vi "dsbsc1.vi"() -> ()   [LabVIEW 2018]
uses:
  <vilib>/express/express analysis/Spectral/Block/exnSpectralBlock spectral measurements RMS poly.vi
  <vilib>/express/express analysis/Spectral/Block/exnSpectralBlock spectral measurements RMS DDT.vi
  <vilib>/express/express analysis/Spectral/XNode/ExpressSpectralMeasurementsBlockNode.xnode
panel:
  out "Waveform Graph 4":dynamicdata(graph)
  out "Waveform Graph 3":dynamicdata(graph)
  out "Waveform Graph 2":dynamicdata(graph)
  out "Waveform Graph":dynamicdata(graph)
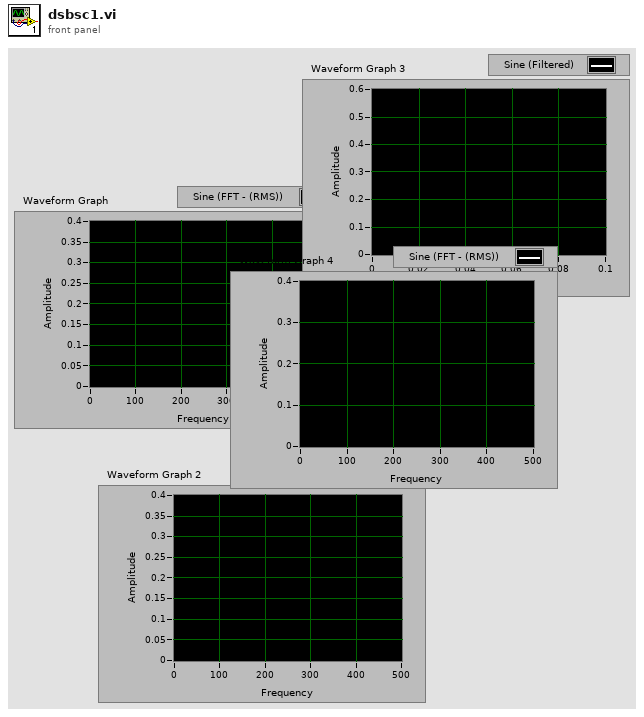
[diagram p1: front panel]
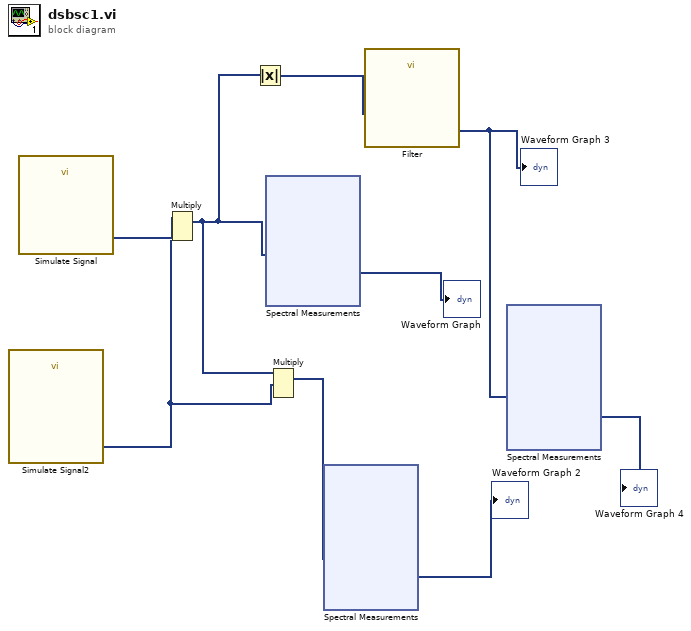
[diagram p0: block diagram]
diagram:
  n1 = call "Simulate Signal2"() -> ("Sine"=w7:dynamicdata)  [unwired: 14 in, 1 out]
  n2 = call "Simulate Signal"() -> ("Sine"=w9:dynamicdata)  [unwired: 14 in, 1 out]
  n3 = Multiply(1:w7, 2:w9) -> (0:w3:dynamicdata)  [unwired: 1 in, 1 out]
  n4 = Absolute Value(x=w3) -> (abs(x)=w4:dynamicdata)
  n5 = xnode "Spectral Measurements"("Signals"=w3) -> ("FFT - (RMS)"=→"Waveform Graph":dynamicdata)  [unwired: 1 in, 2 out]
  n6 = Multiply(1:w7, 2:w3) -> (0:w6:dynamicdata)  [unwired: 1 in, 1 out]
  n7 = xnode "Spectral Measurements"("Signals"=w6) -> ("FFT - (RMS)"=→"Waveform Graph 2":dynamicdata)  [unwired: 1 in, 2 out]
  n8 = call "Filter"("Signal"=w4) -> ("Filtered Signal"=w2:dynamicdata)  [unwired: 9 in, 1 out]
  "Waveform Graph 3" <- w2
  n9 = xnode "Spectral Measurements"("Signals"=w2) -> ("FFT - (RMS)"=→"Waveform Graph 4":dynamicdata)  [unwired: 1 in, 2 out]
